vi "KenbakEngine.vi"(11 "Inputs":T11) -> (0 "Adder":T2, 1 "Clocks And Memory":T3, 2 "Control\nSignals":T7, 3 "States":T10, 4 "Instruction Specific":T1, 5 "K_reg":T6, 6 "W_reg":T4, 7 "I_reg":T5, 8 "L_reg":T8, 9 "T_reg":T9, 10 "Memory":cluster{"MemLo":u8, "MemHi":u8, "Carry?":bool} {"MemHi" format="%x"; "MemLo" format="%x"})   [LabVIEW 2012]
panel:
  out "JS4":bool
  out "JS3":bool
  out "JS2":bool
  out "JS1":bool
  out "JS0":bool
  out "JDL1":bool
  out "JDL0":bool
  out "KP":bool
  out "PF":bool
  out "PT":bool
  out "PO":bool
  out "ED":bool
  out "WD":bool
  out "BM":bool
  out "WT":bool
  out "WL":bool
  out "WJ":bool
  out "WK":bool
  out "CY":bool
  out "OV":bool
  out "OF":bool
  out "CR":bool
  out "SUM":bool
  out "ADD":bool
  out "C":bool
  out "JC":bool
  out "TS":bool
  out "BD":bool
  out "B":bool
  out "A":bool
  out "LONGLOGIC":bool
  out "LS":bool
  out "RR":bool
  out "BT":bool
  out "TX":bool
  out "HF":bool
  out "JW3":bool
  out "JW7":bool
  out "W7":bool
  out "W6":bool
  out "W5":bool
  out "W4":bool
  out "W3":bool
  out "W2":bool
  out "W1":bool
  out "W0":bool
  out "K7":bool
  out "K6":bool
  out "K5":bool
  out "K4":bool
  out "K3":bool
  out "K2":bool
  out "K1":bool
  out "K0":bool
  out "KS":bool
  out "Run":bool
  out "Input":bool
  out "Mem":bool
  out "Add":bool
  out "X4":bool
  out "X3":bool
  out "X2":bool
  out "X1":bool
  out "BU":bool
  out "MR":bool
  out "FT":bool
  out "I4":bool
  out "I5":bool
  out "I6":bool
  out "I7":bool
  out "I3":bool
  out "I2":bool
  out "I1":bool
  out "I0":bool
  out "CL":bool
  out "DA":bool
  out "HT":bool
  out "EA":bool
  out "DD":bool
  out "EN":bool
  out "GO":bool
  out "UT":bool
  out "IN":bool
  out "R":bool
  out "A7":bool
  out "SQ":bool
  out "SP":bool
  out "SW":bool
  out "SC":bool
  out "SD":bool
  out "SZ":bool
  out "SG":bool
  out "SM":bool
  out "SH":bool
  out "SK":bool
  out "SF":bool
  out "SN":bool
  out "SJ":bool
  out "SL":bool
  out "SA":bool
  out "QB":bool
  out "SX":bool
  out "SY":bool
  out "SB":bool
  out "ST":bool
  out "SV":bool
  out "SE":bool
  out "SU":bool
  out "SS":bool
  out "SR":bool
  out "QE":bool
  out "QF":bool
  out "QD":bool
  out "QC":bool
  out "Carry?":bool
  out "/ T7 \\":bool
  out "LC":bool
  out "CM":bool
  out "L7":bool
  out "L6":bool
  out "L5":bool
  out "L4":bool
  out "L3":bool
  out "L2":bool
  out "L1":bool
  out "L0":bool
  out "T7":bool
  out "T6":bool
  out "T5":bool
  out "T4":bool
  out "T3":bool
  out "T2":bool
  out "T1":bool
  out "T0":bool
  out "F1":bool
  out "F2":bool
  out "C7":bool
  out "CP":bool
  out "CT":bool
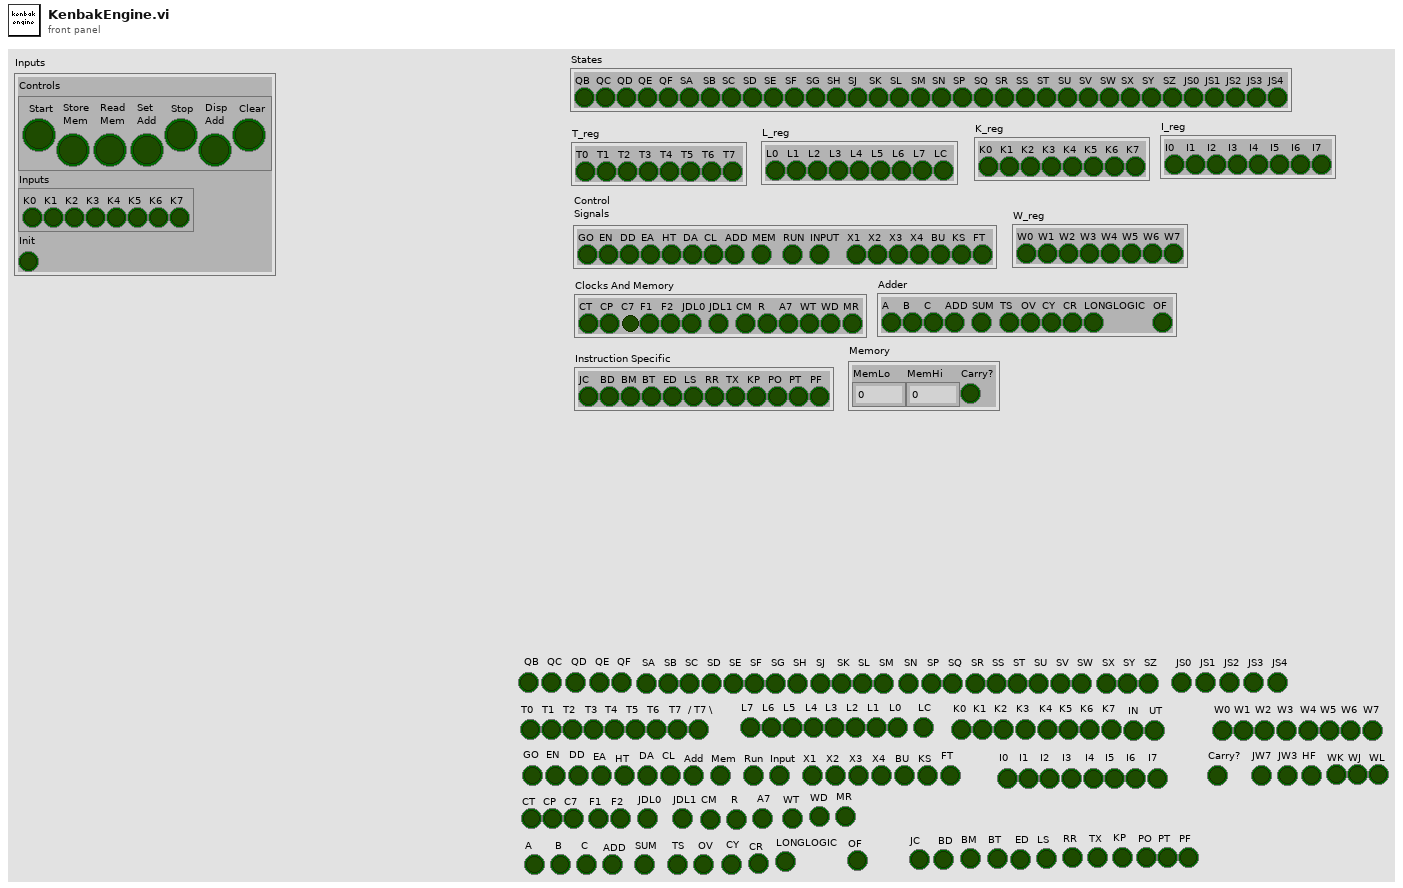
[diagram p1: front panel]
types:
  T1 = cluster{"JC":bool, "BD":bool, "BM":bool, "BT":bool, "ED":bool, "LS":bool, "RR":bool, "TX":bool, "KP":bool, "PO":bool, "PT":bool, "PF":bool}
  T2 = cluster{"A":bool, "B":bool, "C":bool, "ADD":bool, "SUM":bool, "TS":bool, "OV":bool, "CY":bool, "CR":bool, "LONGLOGIC":bool, "OF":bool}
  T3 = cluster{"CT":bool, "CP":bool, "C7":bool, "F1":bool, "F2":bool, "JDL0":bool, "JDL1":bool, "CM":bool, "R":bool, "A7":bool, "WT":bool, "WD":bool, "MR":bool}
  T4 = cluster{"W0":bool, "W1":bool, "W2":bool, "W3":bool, "W4":bool, "W5":bool, "W6":bool, "W7":bool}
  T5 = cluster{"I0":bool, "I1":bool, "I2":bool, "I3":bool, "I4":bool, "I5":bool, "I6":bool, "I7":bool}
  T6 = cluster{"K0":bool, "K1":bool, "K2":bool, "K3":bool, "K4":bool, "K5":bool, "K6":bool, "K7":bool}
  T7 = cluster{"GO":bool, "EN":bool, "DD":bool, "EA":bool, "HT":bool, "DA":bool, "CL":bool, "ADD":bool, "MEM":bool, "RUN":bool, "INPUT":bool, "X1":bool, "X2":bool, "X3":bool, "X4":bool, "BU":bool, "KS":bool, "FT":bool}
  T8 = cluster{"L0":bool, "L1":bool, "L2":bool, "L3":bool, "L4":bool, "L5":bool, "L6":bool, "L7":bool, "LC":bool}
  T9 = cluster{"T0":bool, "T1":bool, "T2":bool, "T3":bool, "T4":bool, "T5":bool, "T6":bool, "T7":bool}
  T10 = cluster{"QB":bool, "QC":bool, "QD":bool, "QE":bool, "QF":bool, "SA":bool, "SB":bool, "SC":bool, "SD":bool, "SE":bool, "SF":bool, "SG":bool, "SH":bool, "SJ":bool, "SK":bool, "SL":bool, "SM":bool, "SN":bool, "SP":bool, "SQ":bool, "SR":bool, "SS":bool, "ST":bool, "SU":bool, "SV":bool, "SW":bool, "SX":bool, "SY":bool, "SZ":bool, "JS0":bool, "JS1":bool, "JS2":bool, "JS3":bool, "JS4":bool}
  T11 = cluster{"Controls":cluster{"Start":bool, "Store\nMem":bool, "Read\nMem":bool, "Set\nAdd":bool, "Stop":bool, "Disp\nAdd":bool, "Clear":bool}, "Inputs":cluster{"K0":bool, "K1":bool, "K2":bool, "K3":bool, "K4":bool, "K5":bool, "K6":bool, "K7":bool}, "Init":bool}
  T12 = cluster{"Start":bool, "Store\nMem":bool, "Read\nMem":bool, "Set\nAdd":bool, "Stop":bool, "Disp\nAdd":bool, "Clear":bool}
  T13 = cluster{"OA":bool, "OB":bool, "OC":bool, "OD":bool, "OA":bool, "OB":bool, "OC":bool, "OD":bool}
  T14 = cluster{"OD":bool, "OC":bool, "OB":bool, "OA":bool, "OD":bool, "OC":bool, "OB":bool, "OA":bool, "Q":bool}
  T15 = cluster{"OA":bool, "OB":bool, "OC":bool, "OD":bool, bool, bool, bool, bool, bool, "0":bool, bool, bool, bool, bool, bool, bool, bool, bool}
  T16 = cluster{"1":bool, "0":bool, "1":bool, "3":bool, "2":bool, "0":bool, "4":bool, "2":bool, "3":bool, "7":bool, "3":bool, "7":bool, "1":bool, "5":bool, "2":bool, "6":bool, "0":bool, "4":bool, "0":bool, "6":bool, "4":bool, "5":bool, "5":bool, "6":bool, "6":bool, "1":bool, "2":bool, "3":bool, "4":bool, "Q":bool, "Q":bool, "Q":bool, "Q":bool, "Q":bool}
  T17 = cluster{"OD":bool, "OC":bool, "OB":bool, "OA":bool, "OD":bool, "OC":bool, "OB":bool, "OA":bool}
  T18 = cluster{bool, bool, "/Q\\":bool, bool, bool, "/Q\\":bool, "Q":bool, "Q":bool, bool, bool, bool}
  T19 = cluster{"Clk":bool, bool, bool, bool, bool, bool, bool, bool, bool, "/Q\\":bool, bool, bool, bool}
  T20 = cluster{bool, "Q":bool, bool, bool, "/Q\\":bool, bool, bool, "OD":bool, bool, "OD":bool, "OC":bool, "OB":bool}
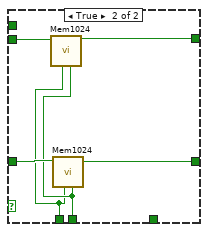
[diagram p2: hidden frame]
diagram:
  w204 = TRUE ("x")
  w226 = FALSE ("Serial\nInput")
  w257 = TRUE ("Set")
  w294 = TRUE ("Set")
  w295 = TRUE ("Set")
  w305 = FALSE ("y")
  w317 = TRUE ("Reset")
  w327 = TRUE ("Set")
  w338 = TRUE ("Set")
  w513 = TRUE ("Set")
  w514 = TRUE ("Set")
  w521 = TRUE ("Set")
  w638 = TRUE ("Set")
  w643 = TRUE ("Set")
  w650 = FALSE ("B")
  w651 = FALSE ("Mode\nControl")
  w654 = TRUE ("Set")
  w657 = FALSE ("B")
  w658 = FALSE ("Mode\nControl")
  w664 = TRUE
  w670 = TRUE ("Set")
  w672 = TRUE ("Set")
  # "JSX  0  1  2  3  4\nQB = 1, 0, 0, 1, 0\nQC = 0, 0, 0, 0, 0\nQD = 1, 0, 0, 0, 0\nQE = 1, 1, 0, 0, 0\nQF = 0, 1, 0, 0, 0\nSA = 0, 0, 0, 1, 0\nSB = 0, 0, 1, 1, 0\nSC = 0, 1, 0, 1, 1\nSD = 1, 1, 0, 1, 1\nSE = 1, 1, 1, 0, 0\nSF = 1, 1, 0, 0, 1\nSG = 1, 1, 1, 0, 1\nSH = 1, 0, 0, 0, 1\nSJ = 1, 0, 1, 0, 1\nSK = 0, 1, 0, 0, 1\nSL = 0, 1, 1, 0, 1\nSM = 0, 0, 0, 0, 1\nSN = 0, 0, 1, 0, 1\nSP = 0, 0, 0, 1, 1\nSQ = 0, 1, 1, 1, 1\nSR = 0, 0, 1, 0, 0\nSS = 1, 0, 1, 0, 0\nST = 1, 0, 1, 1, 0\nSU = 0, 1, 1, 0, 0\nSV = 0, 1, 1, 1, 0\nSW = 1, 0, 0, 1, 1\nSX = 0, 1, 0, 1, 0\nSY = 1, 1, 0, 1, 0\nSZ = 0, 0, 1, 1, 1"
  # "-IN+-BU"
  # "-IN+-CL"
  # "I11"
  # "I10"
  # "I2+-I1+I0"
  # "EN+DD"
  # "JS0"
  # "JS1"
  # "JS2"
  # "JS3"
  # "JS4"
  # "JS0B"
  # "JS0A"
  # "JS1B"
  # "JS2A"
  # "CM"
  # "JS1A"
  # "JS3A"
  # "JS3-4B"
  # "G5"
  # "G4"
  # "G3"
  # "G2"
  # "G1"
  n1 = Unbundle By Name("Inputs") -> ("Controls"=w165:T12)
  n2 = Unbundle By Name("Inputs") -> ("Inputs"=w2:T6)
  n3 = Unbundle By Name(w165) -> ("Start"=w164:bool, "Store\nMem"=w163:bool, "Read\nMem"=w162:bool, "Set\nAdd"=w161:bool, "Stop"=w106:bool, "Disp\nAdd"=w104:bool, "Clear"=w102:bool)
  n4 = Cluster To Array(cluster=w2) -> (array=w1:bool[])
  n5 = call "Clock.vi"("Slices"=u32 2) -> ("Clk"=w67:bool)  [unwired: 10 in]
  "CT" <- w67
  n6 = Index Array(array=w1) -> (element #1=w191:bool, element #2=w190:bool, element #3=w188:bool, element #4=w186:bool, element #5=w184:bool, element #6=w182:bool, element #7=w180:bool, element #8=w177:bool)  [unwired: 8 in]
  n7 = Not And(1:w67, 2:w67) -> (0:w673:bool)
  n8 = feedback #1() -> (w671:bool)  [unwired: 1 in]
  n9 = call "DflipFlop_Fast.vi"("D"=w671, "Clock"=w673, "Reset"=w672, "Set"=w672) -> ("/Q\\"=w175:bool, "Q"=w659:bool)  [unwired: 6 in]
  n10 = feedback-in #1(w175) -> ()
  n11 = Not(x=w182) -> (.not. x?=w181:bool)
  n12 = Not(x=w180) -> (.not. x?=w179:bool)
  n13 = Not(x=w177) -> (.not. x?=w178:bool)
  n14 = Not(x=w191) -> (.not. x?=w192:bool)
  n15 = Not(x=w190) -> (.not. x?=w189:bool)
  n16 = Not(x=w188) -> (.not. x?=w187:bool)
  n17 = Not(x=w186) -> (.not. x?=w185:bool)
  n18 = Not(x=w184) -> (.not. x?=w183:bool)
  n19 = feedback #2() -> (w640:bool)  [unwired: 1 in]
  n20 = Not(x=w106) -> (.not. x?=w105:bool)
  "HT" <- w105
  n21 = Not(x=w164) -> (.not. x?=w520:bool)
  n22 = Not(x=w162) -> (.not. x?=w518:bool)
  n23 = Not(x=w161) -> (.not. x?=w517:bool)
  n24 = Not(x=w104) -> (.not. x?=w103:bool)
  "DA" <- w103
  n25 = Not(x=w102) -> (.not. x?=w101:bool)
  "CL" <- w101
  n26 = Not(x=w163) -> (.not. x?=w519:bool)
  n27 = feedback #3() -> (w667:bool)  [unwired: 1 in]
  n28 = Compound Arithmetic op=AND(w667, w667, w640) -> (w669:bool)
  n29 = Not(x=w669) -> (.not. x?=w668:bool)
  n30 = call "DflipFlop_Fast.vi"("D"=w668, "Clock"=w659, "Reset"=w670, "Set"=w670) -> ("/Q\\"=w663:bool, "Q"=w662:bool)  [unwired: 6 in]
  n31 = feedback-in #3(w662) -> ()
  n32 = Not And(1:w659, 2:w659) -> (0:w661:bool)
  n33 = feedback #4() -> (w9:bool)  [unwired: 1 in]
  n34 = call "ReverseNot.vi"("In"=w9) -> ("~In"=w8:bool)  [unwired: 14 in]
  n35 = Not And(1:w8, 2:w659) -> (0:w660:bool)
  n36 = Not And(1:w8, 2:w8) -> (0:w639:bool)
  "/ T7 \\" <- w639
  n37 = feedback-in #2(w639) -> ()
  n38 = Not(x=w661) -> (.not. x?=w66:bool)
  "CP" <- w66
  n39 = call "7495_Fast2.vi"("Clk 1\nR-Shift"=w66, "Serial\nInput"=w8, "Clk 2\nL-Shift"=w66, "Mode\nControl"=w658, "D"=w658, "C"=w658, "B"=w658, "A"=w658) -> ("OD"=w12:bool, "OC"=w123:bool, "OB"=w124:bool, "OA"=w125:bool)
  "T0" <- w125
  "T1" <- w124
  "T2" <- w123
  "T3" <- w12
  n40 = Not And(1:w192, 2:w125) -> (0:w469:bool)
  n41 = Not And(1:w189, 2:w124) -> (0:w468:bool)
  n42 = Not And(1:w187, 2:w123) -> (0:w467:bool)
  n43 = Not And(1:w185, 2:w12) -> (0:w466:bool)
  n44 = Not(x=w660) -> (.not. x?=w65:bool)
  "C7" <- w65
  n45 = Not And(1:w65, 2:w65) -> (0:w555:bool)
  n46 = call "7495_Fast2.vi"("Clk 1\nR-Shift"=w66, "Serial\nInput"=FALSE ("Serial\nInput"), "Clk 2\nL-Shift"=w66, "Mode\nControl"=w12, "D"=w657, "C"=w657, "B"=w657, "A"=w12) -> ("OD"=w11:bool, "OC"=w120:bool, "OB"=w121:bool, "OA"=w122:bool)
  "T4" <- w122
  "T5" <- w121
  "T6" <- w120
  "T7" <- w11
  n47 = Not And(1:w183, 2:w122) -> (0:w465:bool)
  n48 = call "ReverseNot.vi"("In"=w11) -> ("~In"=w10:bool)  [unwired: 14 in]
  n49 = feedback-in #4(w10) -> ()
  n50 = Not And(1:w65, 2:w65) -> (0:w512:bool)
  n51 = feedback #5() -> (w457:bool)  [unwired: 1 in]
  n52 = feedback #6() -> (w456:bool)  [unwired: 1 in]
  n53 = Not And(1:w181, 2:w121) -> (0:w464:bool)
  n54 = Compound Arithmetic op=AND(w663, w664, w175) -> (w665:bool)
  n55 = Compound Arithmetic op=AND(w664, w175, w662) -> (w666:bool)
  n56 = Not(x=w665) -> (.not. x?=w64:bool)
  "F1" <- w64
  n57 = Not(x=w666) -> (.not. x?=w63:bool)
  "F2" <- w63
  n58 = feedback #7() -> (w511:bool)  [unwired: 1 in]
  n59 = call "DflipFlop_Fast.vi"("D"=w511, "Clock"=w512, "Reset"=w514, "Set"=w514) -> ("Q"=w445:bool)  [unwired: 6 in, 1 out]
  "UT" <- w445
  n60 = Not And(1:w179, 2:w120) -> (0:w463:bool)
  n61 = Exclusive Or(1:w66, 2:TRUE ("x")) -> (0:w642:bool)
  n62 = Not And(1:w178, 2:w11) -> (0:w462:bool)
  n63 = Compound Arithmetic op=AND(w101, w101, w101) -> (w210:bool)
  n64 = Not(x=w210) -> (.not. x?=w209:bool)
  n65 = Compound Arithmetic op=AND(w469, w468, w467, w466, w465, w464, w463, w462) -> (w96:bool)
  "BU" <- w96
  n66 = Not And(1:w96, 2:w96) -> (0:w174:bool)
  n67 = feedback #8() -> (w648:bool)  [unwired: 1 in]
  n68 = Bundle("OA"=w125, "OB"=w124, "OC"=w123, "OD"=w12, "OA"=w122, "OB"=w121, "OC"=w120, "OD"=w11) -> (→"T_reg":T13)  [unwired: 1 in]
  n69 = feedback #9() -> (w4:bool)  [unwired: 1 in]
  n70 = call "ReverseNot.vi"("In"=w4) -> ("~In"=w3:bool)  [unwired: 14 in]
  n71 = Not And(1:w3, 2:w648) -> (0:w653:bool)
  n72 = Not And(1:w639, 2:w653) -> (0:w652:bool)
  n73 = Exclusive Or(1:w3, 2:w648) -> (0:w649:bool)
  n74 = call "7495_Fast2.vi"("Clk 1\nR-Shift"=w66, "Serial\nInput"=w649, "Clk 2\nL-Shift"=w66, "Mode\nControl"=w651, "D"=w651, "C"=w651, "A"=w3) -> ("OD"=w7:bool, "OC"=w115:bool, "OB"=w114:bool, "OA"=w113:bool)  [unwired: 1 in]
  "L7" <- w113
  "L6" <- w114
  "L5" <- w115
  "L4" <- w7
  n75 = call "DflipFlop_Fast.vi"("D"=w652, "Clock"=w642, "Reset"=w654, "Set"=w654) -> ("Q"=w92:bool)  [unwired: 6 in, 1 out]
  "LC" <- w92
  n76 = call "DflipFlop.vi"("D"=w92, "Clock"=w512, "Reset"=w513, "Set"=w513) -> ("Q"=w207:bool)  [unwired: 6 in, 1 out]
  "IN" <- w207
  n77 = call "7495_Fast2.vi"("Clk 1\nR-Shift"=w207, "Serial\nInput"=FALSE ("Serial\nInput"), "Clk 2\nL-Shift"=w207, "Mode\nControl"=TRUE ("Mode\nControl"), "D"=w517, "C"=w518, "B"=w519, "A"=w520) -> ("OD"=w108:bool, "OC"=w109:bool, "OB"=w110:bool, "OA"=w111:bool)
  "GO" <- w111
  "EN" <- w110
  "DD" <- w109
  "EA" <- w108
  n78 = Not And(1:w111, 2:w111) -> (0:w193:bool)
  n79 = Compound Arithmetic op=AND(w103, w109, w457) -> (w460:bool)
  n80 = Compound Arithmetic op=AND(w110, w109, w103, w103) -> (w510:bool)
  n81 = Compound Arithmetic op=AND(w110, w109, w109, w110) -> (w509:bool)
  n82 = Not(x=w460) -> (.not. x?=w455:bool)
  n83 = Not(x=w510) -> (.not. x?=w508:bool)
  n84 = Not(x=w509) -> (.not. x?=w350:bool)
  n85 = feedback-in #7(w207) -> ()
  n86 = Not And(1:w209, 2:w207) -> (0:w208:bool)
  n87 = Not And(1:w96, 2:w207) -> (0:w206:bool)
  n88 = feedback-in #8(w92) -> ()
  n89 = And(x=w11, y=w92) -> (x .and. y?=w16:bool)
  "Carry?" <- w16
  n90 = Not And(1:w108, 2:w108) -> (0:w422:bool)
  n91 = call "7495_Fast2.vi"("Clk 1\nR-Shift"=w66, "Serial\nInput"=w7, "Clk 2\nL-Shift"=w66, "Mode\nControl"=w650, "D"=w66, "C"=w3, "B"=w650, "A"=w650) -> ("OD"=w5:bool, "OC"=w118:bool, "OB"=w117:bool, "OA"=w116:bool)
  "L3" <- w116
  "L2" <- w117
  "L1" <- w118
  "L0" <- w5
  n92 = call "ReverseNot.vi"("In"=w5) -> ("~In"=w6:bool)  [unwired: 14 in]
  n93 = feedback-in #9(w6) -> ()
  n94 = feedback #10() -> (w437:bool)  [unwired: 1 in]
  n95 = feedback #11() -> (w438:bool)  [unwired: 1 in]
  n96 = feedback #12() -> (w439:bool)  [unwired: 1 in]
  n97 = feedback #13() -> (w440:bool)  [unwired: 1 in]
  n98 = feedback #14() -> (w647:bool)  [unwired: 1 in]
  n99 = feedback #15() -> (w500:bool)  [unwired: 1 in]
  n100 = feedback #16() -> (w501:bool)  [unwired: 1 in]
  n101 = feedback #17() -> (w502:bool)  [unwired: 1 in]
  n102 = feedback #18() -> (w503:bool)  [unwired: 1 in]
  n103 = Bundle("OD"=w5, "OC"=w118, "OB"=w117, "OA"=w116, "OD"=w7, "OC"=w115, "OB"=w114, "OA"=w113, "Q"=w92) -> (→"L_reg":T14)  [unwired: 1 in]
  n104 = feedback #19() -> (w444:bool)  [unwired: 1 in]
  n105 = feedback #20() -> (w443:bool)  [unwired: 1 in]
  n106 = feedback #21() -> (w442:bool)  [unwired: 1 in]
  n107 = feedback #22() -> (w441:bool)  [unwired: 1 in]
  n108 = feedback #23() -> (w507:bool)  [unwired: 1 in]
  n109 = feedback #24() -> (w506:bool)  [unwired: 1 in]
  n110 = feedback #25() -> (w505:bool)  [unwired: 1 in]
  n111 = feedback #26() -> (w504:bool)  [unwired: 1 in]
  n112 = Not And(1:w125, 2:w125) -> (0:w379:bool)
  n113 = Not And(1:w122, 2:w122) -> (0:w369:bool)
  n114 = feedback #27() -> (w381:bool)  [unwired: 1 in]
  n115 = feedback #28() -> (w554:bool)  [unwired: 1 in]
  n116 = call "DflipFlop_Fast.vi"("D"=w554, "Clock"=w555, "Reset"=w638, "Set"=w638) -> ("Q"=w131:bool)  [unwired: 6 in, 1 out]
  "JS0" <- w131
  n117 = feedback #29() -> (w553:bool)  [unwired: 1 in]
  n118 = call "DflipFlop_Fast.vi"("D"=w553, "Clock"=w555, "Reset"=w638, "Set"=w638) -> ("Q"=w130:bool)  [unwired: 6 in, 1 out]
  "JS1" <- w130
  n119 = feedback #30() -> (w552:bool)  [unwired: 1 in]
  n120 = call "DflipFlop_Fast.vi"("D"=w552, "Clock"=w555, "Reset"=w638, "Set"=w638) -> ("Q"=w129:bool)  [unwired: 6 in, 1 out]
  "JS2" <- w129
  n121 = feedback #31() -> (w551:bool)  [unwired: 1 in]
  n122 = call "DflipFlop_Fast.vi"("D"=w551, "Clock"=w555, "Reset"=w638, "Set"=w638) -> ("/Q\\"=w636:bool, "Q"=w128:bool)  [unwired: 6 in]
  "JS3" <- w128
  n123 = feedback #32() -> (w550:bool)  [unwired: 1 in]
  n124 = call "DflipFlop_Fast.vi"("D"=w550, "Clock"=w555, "Reset"=w638, "Set"=w638) -> ("/Q\\"=w637:bool, "Q"=w127:bool)  [unwired: 6 in]
  "JS4" <- w127
  n125 = Not And(1:w637, 2:w636) -> (0:w632:bool)
  n126 = Not And(1:w637, 2:w128) -> (0:w633:bool)
  n127 = Not And(1:w127, 2:w636) -> (0:w634:bool)
  n128 = Not And(1:w127, 2:w128) -> (0:w635:bool)
  n129 = call "7442.vi"("D"=w635, "C"=w129, "B"=w130, "A"=w131) -> ("0"=w142:bool, "1"=w135:bool, "2"=w153:bool, "3"=w152:bool, "4"=w132:bool, "6"=w141:bool)  [unwired: 2 in, 4 out]
  "SP" <- w142
  "SW" <- w135
  "SC" <- w153
  "SD" <- w152
  "SZ" <- w132
  "SQ" <- w141
  n130 = call "7442.vi"("D"=w632, "C"=w129, "B"=w130, "A"=w131) -> ("0"=w107:bool, "1"=w158:bool, "2"=w156:bool, "3"=w157:bool, "4"=w139:bool, "5"=w140:bool, "6"=w137:bool, "7"=w151:bool)  [unwired: 2 in, 2 out]
  "QC" <- w107
  "QD" <- w158
  "QF" <- w156
  "QE" <- w157
  "SR" <- w139
  "SS" <- w140
  "SU" <- w137
  "SE" <- w151
  "Run" <- w107
  n131 = call "7442.vi"("D"=w633, "C"=w129, "B"=w130, "A"=w131) -> ("0"=w155:bool, "1"=w159:bool, "2"=w134:bool, "3"=w133:bool, "4"=w154:bool, "5"=w138:bool, "6"=w136:bool)  [unwired: 2 in, 3 out]
  "SA" <- w155
  "QB" <- w159
  "SX" <- w134
  "SY" <- w133
  "SB" <- w154
  "ST" <- w138
  "SV" <- w136
  n132 = Compound Arithmetic op=AND(w455, w155, w101, w174) -> (w461:bool)
  n133 = Compound Arithmetic op=AND(w103, w155, w456) -> (w459:bool)
  n134 = Not(x=w461) -> (.not. x?=w453:bool)
  n135 = feedback-in #5(w453) -> ()
  n136 = Not(x=w459) -> (.not. x?=w454:bool)
  n137 = Compound Arithmetic op=AND(w454, w109, w101, w174) -> (w458:bool)
  n138 = Not(x=w458) -> (.not. x?=w452:bool)
  n139 = feedback-in #6(w452) -> ()
  n140 = And(x=w454, y=w455) -> (x .and. y?=w100:bool)
  "X1" <- w100
  "Add" <- w100
  n141 = And(x=w455, y=w452) -> (x .and. y?=w99:bool)
  "X2" <- w99
  "Mem" <- w99
  n142 = And(x=w454, y=w453) -> (x .and. y?=w98:bool)
  "X3" <- w98
  n143 = And(x=w453, y=w452) -> (x .and. y?=w97:bool)
  "X4" <- w97
  "Input" <- w97
  n144 = call "7442.vi"("D"=w634, "C"=w129, "B"=w130, "A"=w131) -> ("0"=w144:bool, "1"=w148:bool, "2"=w146:bool, "3"=w150:bool, "4"=w143:bool, "5"=w147:bool, "6"=w145:bool, "7"=w149:bool)  [unwired: 2 in, 2 out]
  "SM" <- w144
  "SH" <- w148
  "SK" <- w146
  "SF" <- w150
  "SN" <- w143
  "SJ" <- w147
  "SL" <- w145
  "SG" <- w149
  n145 = Not And(1:w157, 2:w157) -> (0:w446:bool)
  n146 = And(x=w446, y=w99) -> (x .and. y?=w447:bool)
  n147 = And(x=w446, y=w100) -> (x .and. y?=w448:bool)
  n148 = And(x=w207, y=w97) -> (x .and. y?=w449:bool)
  n149 = And(x=w98, y=w445) -> (x .and. y?=w450:bool)
  n150 = Compound Arithmetic op=OR(w447, w448, w449, w450) -> (w451:bool)
  n151 = Not(x=w451) -> (.not. x?=w95:bool)
  "KS" <- w95
  n152 = Not And(1:w107, 2:w107) -> (0:w498:bool)
  n153 = Not And(1:w207, 2:w498) -> (0:w424:bool)
  n154 = Not And(1:w424, 2:w424) -> (0:w423:bool)
  n155 = Compound Arithmetic op=AND(w152, w141, w157, w140, w424, w424, w142, w157) -> (w499:bool)
  n156 = Not(x=w499) -> (.not. x?=w94:bool)
  "FT" <- w94
  n157 = Bundle("OA"=w111, "OB"=w110, "OC"=w109, "OD"=w108, w105, w103, w101, w100, w99, "0"=w107, w97, w100, w99, w98, w97, w96, w95, w94) -> (→"Control\nSignals":T15)  [unwired: 1 in]
  n158 = Not And(1:w422, 2:w423) -> (0:w421:bool)
  n159 = Not And(1:w94, 2:w94) -> (0:w172:bool)
  n160 = Bundle("1"=w159, "0"=w107, "1"=w158, "3"=w157, "2"=w156, "0"=w155, "4"=w154, "2"=w153, "3"=w152, "7"=w151, "3"=w150, "7"=w149, "1"=w148, "5"=w147, "2"=w146, "6"=w145, "0"=w144, "4"=w143, "0"=w142, "6"=w141, "4"=w139, "5"=w140, "5"=w138, "6"=w137, "6"=w136, "1"=w135, "2"=w134, "3"=w133, "4"=w132, "Q"=w131, "Q"=w130, "Q"=w129, "Q"=w128, "Q"=w127) -> (→"States":T16)  [unwired: 1 in]
  n161 = Not(x=w144) -> (.not. x?=w195:bool)
  n162 = Not(x=w158) -> (.not. x?=w611:bool)
  n163 = Not(x=w154) -> (.not. x?=w630:bool)
  n164 = Not(x=w138) -> (.not. x?=w196:bool)
  n165 = Not(x=w145) -> (.not. x?=w263:bool)
  n166 = Not And(1:w151, 2:w151) -> (0:w352:bool)
  n167 = Not And(1:w156, 2:w156) -> (0:w610:bool)
  n168 = Not And(1:w149, 2:w149) -> (0:w194:bool)
  n169 = Not And(1:w107, 2:w107) -> (0:w544:bool)
  n170 = Not And(1:w132, 2:w132) -> (0:w623:bool)
  n171 = Not And(1:w136, 2:w136) -> (0:w253:bool)
  n172 = Compound Arithmetic op=AND(w152, w152, w137, w137) -> (w628:bool)
  n173 = Not(x=w628) -> (.not. x?=w627:bool)
  n174 = Not And(1:w627, 2:w627) -> (0:w564:bool)
  n175 = Not And(1:w137, 2:w134) -> (0:w532:bool)
  n176 = And(x=w193, y=w544) -> (x .and. y?=w621:bool)
  n177 = Not And(1:w144, 2:w144) -> (0:w529:bool)
  n178 = feedback #33() -> (w378:bool)  [unwired: 1 in]
  n179 = Not And(1:w378, 2:w379) -> (0:w377:bool)
  n180 = Not And(1:w369, 2:w377) -> (0:w376:bool)
  n181 = feedback-in #33(w376) -> ()
  n182 = feedback #34() -> (w387:bool)  [unwired: 1 in]
  n183 = And(x=w610, y=w508) -> (x .and. y?=w614:bool)
  n184 = Compound Arithmetic op=AND(w147, w144, w151, w149) -> (w583:bool)
  n185 = Compound Arithmetic op=AND(w152, w153, w150, w158, w139, w146, w146, w139) -> (w534:bool)
  n186 = Not(x=w583) -> (.not. x?=w582:bool)
  n187 = Not(x=w534) -> (.not. x?=w524:bool)
  n188 = Not And(1:w135, 2:w135) -> (0:w400:bool)
  n189 = Not And(1:w582, 2:w582) -> (0:w584:bool)
  n190 = Not And(1:w107, 2:w107) -> (0:w523:bool)
  n191 = And(x=w107, y=FALSE) -> (x .and. y?=w541:bool)
  n192 = Compound Arithmetic op=AND(w157, w151, w154, w149, w145, w136, w421, w147) -> (w425:bool)
  n193 = Not And(1:w152, 2:w152) -> (0:w248:bool)
  n194 = Not And(1:w159, 2:w159) -> (0:w593:bool)
  n195 = And(x=w523, y=w523) -> (x .and. y?=w526:bool)
  n196 = Not(x=w425) -> (.not. x?=w414:bool)
  n197 = feedback #35() -> (w371:bool)  [unwired: 1 in]
  n198 = And(x=w593, y=w193) -> (x .and. y?=w594:bool)
  n199 = And(x=w544, y=w508) -> (x .and. y?=w597:bool)
  n200 = Not And(1:w193, 2:w544) -> (0:w590:bool)
  n201 = Not And(1:w414, 2:w414) -> (0:w417:bool)
  n202 = Compound Arithmetic op=AND(w140, w133, w136, w143, w143, w132, w132, w132) -> (w578:bool)
  n203 = Not(x=w578) -> (.not. x?=w577:bool)
  n204 = Not And(1:w66, 2:w66) -> (0:w313:bool)
  n205 = Not And(1:w11, 2:w11) -> (0:w316:bool)
  n206 = Not And(1:w577, 2:w577) -> (0:w576:bool)
  n207 = Not And(1:w65, 2:w65) -> (0:w293:bool)
  n208 = Compound Arithmetic op=AND(w148, w146, w150, w155) -> (w572:bool)
  n209 = Not(x=w572) -> (.not. x?=w571:bool)
  n210 = feedback #36() -> (w335:bool)  [unwired: 1 in]
  n211 = Compound Arithmetic op=AND(w139, w134, w153, w153) -> (w543:bool)
  n212 = Not(x=w543) -> (.not. x?=w561:bool)
  n213 = feedback #37() -> (w394:bool)  [unwired: 1 in]
  n214 = feedback #38() -> (w426:bool)  [unwired: 1 in]
  n215 = feedback #39() -> (w427:bool)  [unwired: 1 in]
  n216 = feedback #40() -> (w395:bool)  [unwired: 1 in]
  n217 = Not And(1:w157, 2:w157) -> (0:w351:bool)
  n218 = feedback #41() -> (w430:bool)  [unwired: 1 in]
  n219 = feedback #42() -> (w429:bool)  [unwired: 1 in]
  n220 = feedback #43() -> (w428:bool)  [unwired: 1 in]
  n221 = feedback #44() -> (w393:bool)  [unwired: 1 in]
  n222 = And(x=w100, y=w393) -> (x .and. y?=w436:bool)
  n223 = And(x=w393, y=w524) -> (x .and. y?=w528:bool)
  n224 = And(x=w524, y=w393) -> (x .and. y?=w525:bool)
  n225 = Not Or(1:w526, 2:w525) -> (0:w522:bool)
  n226 = call "DflipFlop_Fast.vi"("D"=w522, "Clock"=w65, "Reset"=w521, "Set"=w521) -> ("/Q\\"=w58:bool, "Q"=w171:bool)  [unwired: 6 in]
  "A7" <- w58
  n227 = Not And(1:w151, 2:w151) -> (0:w353:bool)
  n228 = Not And(1:w143, 2:w143) -> (0:w283:bool)
  n229 = Not And(1:w350, 2:w351) -> (0:w347:bool)
  n230 = Not And(1:w154, 2:w154) -> (0:w341:bool)
  n231 = Not And(1:w141, 2:w141) -> (0:w339:bool)
  n232 = Not And(1:w11, 2:w11) -> (0:w315:bool)
  n233 = And(x=w124, y=w339) -> (x .and. y?=w357:bool)
  n234 = Not And(1:w105, 2:w105) -> (0:w167:bool)
  n235 = Not And(1:w141, 2:w133) -> (0:w287:bool)
  n236 = Not And(1:w110, 2:w110) -> (0:w280:bool)
  n237 = Not And(1:w157, 2:w157) -> (0:w279:bool)
  n238 = Not And(1:w287, 2:w287) -> (0:w284:bool)
  n239 = Not And(1:w280, 2:w279) -> (0:w278:bool)
  n240 = Not And(1:w278, 2:w140) -> (0:w259:bool)
  "WL" <- w259
  n241 = And(x=w259, y=w259) -> (x .and. y?=w275:bool)
  n242 = Not And(1:TRUE ("y"), 2:w66) -> (0:w245:bool)
  n243 = feedback #45() -> (w311:bool)  [unwired: 1 in]
  n244 = call "7495_Fast2.vi"("Clk 1\nR-Shift"=w66, "Serial\nInput"=w311, "Clk 2\nL-Shift"=w66, "Mode\nControl"=w172, "D"=w503, "C"=w502, "B"=w501, "A"=w500) -> ("OD"=w15:bool, "OC"=w80:bool, "OB"=w79:bool, "OA"=w78:bool)
  "I4" <- w15
  "I5" <- w80
  "I6" <- w79
  "I7" <- w78
  n245 = feedback-in #15(w78) -> ()
  n246 = feedback-in #16(w79) -> ()
  n247 = feedback-in #17(w80) -> ()
  n248 = feedback-in #18(w15) -> ()
  n249 = call "7495_Fast2.vi"("Clk 1\nR-Shift"=w66, "Serial\nInput"=w15, "Clk 2\nL-Shift"=w66, "Mode\nControl"=w172, "D"=w504, "C"=w505, "B"=w506, "A"=w507) -> ("OD"=w84:bool, "OC"=w83:bool, "OB"=w82:bool, "OA"=w81:bool)
  "I0" <- w84
  "I1" <- w83
  "I2" <- w82
  "I3" <- w81
  n250 = feedback-in #23(w81) -> ()
  n251 = feedback-in #24(w82) -> ()
  n252 = feedback-in #25(w83) -> ()
  n253 = feedback-in #26(w84) -> ()
  n254 = Not(x=w80) -> (.not. x?=w282:bool)
  n255 = Not And(1:w15, 2:w15) -> (0:w492:bool)
  n256 = Not(x=w84) -> (.not. x?=w485:bool)
  n257 = Not And(1:w82, 2:w82) -> (0:w484:bool)
  n258 = Compound Arithmetic op=AND(w484, w485, w83) -> (w491:bool)
  n259 = Not And(1:w84, 2:w253) -> (0:w557:bool)
  n260 = Not(x=w491) -> (.not. x?=w267:bool)
  n261 = Not And(1:w263, 2:w267) -> (0:w581:bool)
  n262 = Not And(1:w263, 2:w581) -> (0:w574:bool)
  n263 = Not And(1:w83, 2:w83) -> (0:w481:bool)
  n264 = Not And(1:w84, 2:w84) -> (0:w480:bool)
  n265 = Not(x=w79) -> (.not. x?=w239:bool)
  n266 = Not And(1:w79, 2:w78) -> (0:w366:bool)
  n267 = Not And(1:w81, 2:w15) -> (0:w389:bool)
  n268 = Not And(1:w78, 2:w78) -> (0:w266:bool)
  n269 = Not And(1:w282, 2:w282) -> (0:w486:bool)
  n270 = Not And(1:w480, 2:w481) -> (0:w482:bool)
  n271 = Not(x=w366) -> (.not. x?=w495:bool)
  n272 = Not(x=w366) -> (.not. x?=w290:bool)
  n273 = Not And(1:w82, 2:w82) -> (0:w365:bool)
  n274 = Not And(1:w81, 2:w81) -> (0:w388:bool)
  n275 = Not And(1:w495, 2:w389) -> (0:w349:bool)
  n276 = Not(x=w389) -> (.not. x?=w494:bool)
  n277 = Compound Arithmetic op=AND(w282, w84, w82) -> (w488:bool)
  n278 = Compound Arithmetic op=AND(w482, w282, w82) -> (w483:bool)
  n279 = Compound Arithmetic op=AND(w267, w486, w81) -> (w487:bool)
  n280 = Not And(1:w388, 2:w365) -> (0:w493:bool)
  n281 = Not And(1:w81, 2:w15) -> (0:w322:bool)
  n282 = Not And(1:w388, 2:w15) -> (0:w392:bool)
  n283 = Not And(1:w81, 2:w389) -> (0:w391:bool)
  n284 = Not And(1:w388, 2:w389) -> (0:w390:bool)
  n285 = Not And(1:w366, 2:w78) -> (0:w496:bool)
  n286 = Not And(1:w79, 2:w366) -> (0:w497:bool)
  n287 = Not(x=w488) -> (.not. x?=w476:bool)
  n288 = Not(x=w483) -> (.not. x?=w473:bool)
  n289 = Not(x=w487) -> (.not. x?=w475:bool)
  n290 = Not And(1:w494, 2:w366) -> (0:w489:bool)
  n291 = Not And(1:w489, 2:w282) -> (0:w603:bool)
  n292 = Compound Arithmetic op=AND(w489, w481, w282, w82) -> (w490:bool)
  n293 = Not(x=w490) -> (.not. x?=w477:bool)
  n294 = Not(x=w496) -> ()  [unwired: 1 out]
  n295 = Not(x=w497) -> (.not. x?=w472:bool)
  n296 = Not And(1:w489, 2:w489) -> (0:w169:bool)
  n297 = Not And(1:w169, 2:w282) -> (0:w545:bool)
  n298 = call "7495_Fast2.vi"("Clk 1\nR-Shift"=w66, "Serial\nInput"=w387, "Clk 2\nL-Shift"=w66, "Mode\nControl"=w11, "D"=w390, "C"=w391, "B"=w392, "A"=w322) -> ("OD"=w34:bool)  [unwired: 3 out]
  "TX" <- w34
  n299 = Compound Arithmetic op=AND(w477, w267, w476, w475) -> (w478:bool)
  n300 = Not(x=w282) -> (.not. x?=w479:bool)
  n301 = Not And(1:w473, 2:w475) -> (0:w168:bool)
  n302 = Not(x=w478) -> (.not. x?=w474:bool)
  n303 = feedback-in #34(w34) -> ()
  n304 = Compound Arithmetic op=AND(w194, w282, w481) -> (w600:bool)
  n305 = Not And(1:w34, 2:w34) -> (0:w372:bool)
  n306 = Compound Arithmetic op=AND(w372, w379, w372) -> (w386:bool)
  n307 = Not(x=w386) -> (.not. x?=w382:bool)
  n308 = Not And(1:w381, 2:w382) -> (0:w35:bool)
  "RR" <- w35
  n309 = Not And(1:w379, 2:w35) -> (0:w380:bool)
  n310 = feedback-in #27(w380) -> ()
  n311 = Not And(1:w80, 2:w80) -> (0:w323:bool)
  n312 = Not And(1:w529, 2:w472) -> (0:w531:bool)
  n313 = Not And(1:w479, 2:w532) -> (0:w533:bool)
  n314 = Not And(1:w472, 2:w529) -> (0:w530:bool)
  n315 = Not(x=w600) -> (.not. x?=w599:bool)
  n316 = And(x=w352, y=w474) -> (x .and. y?=w616:bool)
  n317 = Not And(1:w599, 2:w147) -> (0:w601:bool)
  n318 = Compound Arithmetic op=AND(w323, w372, w377) -> (w385:bool)
  n319 = Compound Arithmetic op=AND(w376, w372, w80) -> (w384:bool)
  n320 = Compound Arithmetic op=AND(w155, w148, w530, w138) -> (w536:bool)
  n321 = Compound Arithmetic op=AND(w155, w533, w531, w138) -> (w538:bool)
  n322 = Not(x=w385) -> (.not. x?=w374:bool)
  n323 = Not(x=w384) -> (.not. x?=w375:bool)
  n324 = Not(x=w536) -> (.not. x?=w535:bool)
  n325 = Not(x=w538) -> (.not. x?=w537:bool)
  n326 = Not And(1:w601, 2:w489) -> (0:w566:bool)
  n327 = Not(x=w78) -> (.not. x?=w403:bool)
  n328 = Compound Arithmetic op=AND(w372, w372, w369) -> (w373:bool)
  n329 = Compound Arithmetic op=AND(w374, w375, w375) -> (w383:bool)
  n330 = Not(x=w373) -> (.not. x?=w368:bool)
  n331 = And(x=w537, y=w125) -> (x .and. y?=w542:bool)
  n332 = And(x=w124, y=w535) -> (x .and. y?=w540:bool)
  n333 = Not(x=w383) -> (.not. x?=w38:bool)
  "BT" <- w38
  n334 = Compound Arithmetic op=AND(w400, w239, w403) -> (w420:bool)
  n335 = Not(x=w420) -> (.not. x?=w416:bool)
  n336 = Compound Arithmetic op=AND(w194, w481, w282) -> (w587:bool)
  n337 = Compound Arithmetic op=OR(w542, w541, w540, w528) -> (w539:bool)
  n338 = Not And(1:w35, 2:w35) -> (0:w404:bool)
  n339 = Not And(1:w371, 2:w368) -> (0:w370:bool)
  n340 = Not And(1:w369, 2:w370) -> (0:w36:bool)
  "LS" <- w36
  n341 = Compound Arithmetic op=AND(w78, w239, w36) -> (w419:bool)
  n342 = Not(x=w419) -> (.not. x?=w408:bool)
  n343 = feedback-in #35(w36) -> ()
  n344 = Not(x=w587) -> (.not. x?=w586:bool)
  n345 = And(x=w168, y=w352) -> (x .and. y?=w595:bool)
  n346 = And(x=w248, y=w493) -> (x .and. y?=w596:bool)
  n347 = Not(x=w539) -> (.not. x?=w59:bool)
  "R" <- w59
  n348 = Exclusive Or(1:w3, 2:w59) -> (0:w641:bool)
  n349 = Not And(1:w641, 2:w647) -> (0:w644:bool)
  n350 = Not And(1:w639, 2:w644) -> (0:w645:bool)
  n351 = call "DflipFlop_Fast.vi"("D"=w645, "Clock"=w642, "Reset"=w643, "Set"=w643) -> ("/Q\\"=w197:bool, "Q"=w646:bool)  [unwired: 6 in]
  n352 = feedback-in #14(w646) -> ()
  n353 = Not And(1:w197, 2:w197) -> (0:w60:bool)
  "CM" <- w60
  n354 = Compound Arithmetic op=AND(w60, w60, w60) -> (w617:bool)
  n355 = Not(x=w617) -> (.not. x?=w588:bool)
  n356 = Not And(1:w60, 2:w603) -> (0:w604:bool)
  n357 = Compound Arithmetic op=AND(w492, w60, w492) -> (w606:bool)
  n358 = Not And(1:w604, 2:w604) -> (0:w602:bool)
  n359 = Not(x=w606) -> (.not. x?=w605:bool)
  n360 = And(x=w532, y=w60) -> (x .and. y?=w618:bool)
  n361 = And(x=w195, y=w602) -> (x .and. y?=w619:bool)
  n362 = And(x=w605, y=w196) -> (x .and. y?=w620:bool)
  n363 = Not And(1:w60, 2:w196) -> (0:w580:bool)
  n364 = Not And(1:w60, 2:w196) -> (0:w608:bool)
  n365 = Compound Arithmetic op=OR(w618, w619, w620, w621) -> (w622:bool)
  n366 = Not And(1:w608, 2:w608) -> (0:w609:bool)
  n367 = Not(x=w622) -> (.not. x?=w575:bool)
  n368 = Compound Arithmetic op=AND(w195, w60, w545) -> (w607:bool)
  n369 = And(x=w611, y=w60) -> (x .and. y?=w615:bool)
  n370 = And(x=w15, y=w609) -> (x .and. y?=w613:bool)
  n371 = Not(x=w607) -> (.not. x?=w569:bool)
  n372 = Compound Arithmetic op=OR(w616, w615, w614, w613) -> (w612:bool)
  n373 = Not(x=w612) -> (.not. x?=w567:bool)
  n374 = Not And(1:w588, 2:w196) -> (0:w589:bool)
  n375 = Compound Arithmetic op=AND(w408, w408, w408) -> (w409:bool)
  n376 = Not And(1:w403, 2:w404) -> (0:w401:bool)
  n377 = Not And(1:w78, 2:w35) -> (0:w252:bool)
  n378 = Not And(1:w416, 2:w416) -> (0:w415:bool)
  n379 = Compound Arithmetic op=OR(w594, w595, w596, w597) -> (w598:bool)
  n380 = Not(x=w409) -> (.not. x?=w407:bool)
  n381 = Compound Arithmetic op=AND(w590, w586, w589) -> (w592:bool)
  n382 = Not(x=w592) -> (.not. x?=w591:bool)
  n383 = Not(x=w598) -> (.not. x?=w560:bool)
  n384 = Compound Arithmetic op=AND(w417, w416, w393) -> (w418:bool)
  n385 = Not And(1:w415, 2:w394) -> (0:w410:bool)
  n386 = Compound Arithmetic op=AND(w252, w401, w400) -> (w402:bool)
  n387 = Bundle("OD"=w84, "OC"=w83, "OB"=w82, "OA"=w81, "OD"=w15, "OC"=w80, "OB"=w79, "OA"=w78) -> (→"I_reg":T17)  [unwired: 1 in]
  n388 = Not And(1:w400, 2:w407) -> (0:w406:bool)
  n389 = Not And(1:w414, 2:w311) -> (0:w411:bool)
  n390 = Not And(1:w79, 2:w78) -> (0:w324:bool)
  n391 = Not(x=w418) -> (.not. x?=w412:bool)
  n392 = Not(x=w402) -> (.not. x?=w399:bool)
  n393 = Not And(1:w591, 2:w591) -> (0:w559:bool)
  n394 = Not And(1:w406, 2:w395) -> (0:w405:bool)
  n395 = Compound Arithmetic op=AND(w323, w322, w324, w283) -> (w326:bool)
  n396 = Not And(1:w399, 2:w399) -> (0:w396:bool)
  "HF" <- w396
  n397 = Compound Arithmetic op=AND(w412, w411, w410) -> (w413:bool)
  n398 = Not(x=w326) -> (.not. x?=w325:bool)
  n399 = Not And(1:w405, 2:w405) -> (0:w397:bool)
  "JW3" <- w397
  n400 = Not(x=w413) -> (.not. x?=w398:bool)
  "JW7" <- w398
  n401 = call "DflipFlop_Fast.vi"("D"=w325, "Clock"=w293, "Reset"=w327, "Set"=w327) -> ("/Q\\"=w48:bool, "Q"=w176:bool)  [unwired: 6 in]
  "TS" <- w48
  n402 = Not And(1:w571, 2:w60) -> (0:w570:bool)
  n403 = Not And(1:w561, 2:w60) -> (0:w558:bool)
  n404 = Not And(1:w83, 2:w83) -> (0:w319:bool)
  n405 = call "7495_Fast2.vi"("Clk 1\nR-Shift"=w66, "Serial\nInput"=w398, "Clk 2\nL-Shift"=w66, "Mode\nControl"=w396, "D"=w395, "C"=w427, "B"=w426, "A"=w394) -> ("OD"=w72:bool, "OC"=w71:bool, "OB"=w70:bool, "OA"=w69:bool)
  "W4" <- w72
  "W5" <- w71
  "W6" <- w70
  "W7" <- w69
  n406 = feedback-in #37(w69) -> ()
  n407 = feedback-in #38(w70) -> ()
  n408 = feedback-in #39(w71) -> ()
  n409 = feedback-in #40(w72) -> ()
  n410 = Compound Arithmetic op=AND(w83, w366, w282, w365, w366, w84, w15, w81) -> (w367:bool)
  n411 = Not And(1:w84, 2:w84) -> (0:w249:bool)
  n412 = Not And(1:w319, 2:w84) -> (0:w318:bool)
  n413 = Not(x=w367) -> (.not. x?=w364:bool)
  n414 = Not(x=w364) -> (.not. x?=w44:bool)
  "LONGLOGIC" <- w44
  n415 = call "7495_Fast2.vi"("Clk 1\nR-Shift"=w66, "Serial\nInput"=w397, "Clk 2\nL-Shift"=w66, "Mode\nControl"=w396, "D"=w393, "C"=w428, "B"=w429, "A"=w430) -> ("OD"=w76:bool, "OC"=w75:bool, "OB"=w74:bool, "OA"=w73:bool)
  "W0" <- w76
  "W1" <- w75
  "W2" <- w74
  "W3" <- w73
  n416 = feedback-in #41(w73) -> ()
  n417 = feedback-in #42(w74) -> ()
  n418 = feedback-in #43(w75) -> ()
  n419 = feedback-in #44(w76) -> ()
  n420 = Not And(1:w349, 2:w283) -> (0:w348:bool)
  n421 = Not And(1:w353, 2:w44) -> (0:w346:bool)
  n422 = Not(x=w81) -> (.not. x?=w289:bool)
  n423 = Not And(1:w347, 2:w346) -> (0:w340:bool)
  n424 = Not And(1:w348, 2:w147) -> (0:w342:bool)
  n425 = Not And(1:w346, 2:w157) -> (0:w344:bool)
  n426 = Not And(1:w15, 2:w283) -> (0:w354:bool)
  n427 = Compound Arithmetic op=AND(w344, w344, w344) -> (w363:bool)
  n428 = Not And(1:w267, 2:w267) -> (0:w264:bool)
  n429 = Not(x=w363) -> (.not. x?=w345:bool)
  n430 = Compound Arithmetic op=AND(w264, w38, w263) -> (w265:bool)
  n431 = Not(x=w265) -> (.not. x?=w262:bool)
  n432 = And(x=w125, y=w340) -> (x .and. y?=w359:bool)
  n433 = And(x=w76, y=w342) -> (x .and. y?=w358:bool)
  n434 = Compound Arithmetic op=AND(w76, w344, w344) -> (w361:bool)
  n435 = Not And(1:w262, 2:w262) -> (0:w39:bool)
  "BM" <- w39
  n436 = Not(x=w361) -> (.not. x?=w343:bool)
  n437 = Compound Arithmetic op=AND(w253, w252, w249) -> (w255:bool)
  n438 = And(x=w39, y=w266) -> (x .and. y?=w276:bool)
  n439 = And(x=w259, y=w84) -> (x .and. y?=w269:bool)
  n440 = And(x=w79, y=w39) -> (x .and. y?=w271:bool)
  n441 = Not(x=w255) -> (.not. x?=w251:bool)
  n442 = Compound Arithmetic op=AND(w251, w248, w167) -> (w254:bool)
  n443 = Not(x=w254) -> (.not. x?=w250:bool)
  n444 = Bundle("OD"=w76, "OC"=w75, "OB"=w74, "OA"=w73, "OD"=w72, "OC"=w71, "OB"=w70, "OA"=w69) -> (→"W_reg":T17)  [unwired: 1 in]
  n445 = Not And(1:w283, 2:w282) -> (0:w281:bool)
  n446 = Not And(1:w281, 2:w154) -> (0:w260:bool)
  "WJ" <- w260
  n447 = And(x=w260, y=w260) -> (x .and. y?=w274:bool)
  n448 = Not And(1:w81, 2:w283) -> (0:w50:bool)
  "ADD" <- w50
  n449 = feedback #46() -> (w242:bool)  [unwired: 1 in]
  n450 = Compound Arithmetic op=AND(w242, w251, w250) -> (w256:bool)
  n451 = Not(x=w256) -> (.not. x?=w246:bool)
  n452 = Compound Arithmetic op=AND(w107, w107, w246) -> (w247:bool)
  n453 = Not(x=w247) -> (.not. x?=w244:bool)
  n454 = call "DflipFlop_Fast.vi"("D"=w244, "Clock"=w245, "Reset"=w257, "Set"=w257) -> ("/Q\\"=w37:bool, "Q"=w199:bool)  [unwired: 6 in]
  "ED" <- w37
  n455 = Not And(1:w199, 2:w630) -> (0:w625:bool)
  n456 = Compound Arithmetic op=AND(w625, w153, w135, w134) -> (w626:bool)
  n457 = Compound Arithmetic op=AND(w146, w150, w153, w625) -> (w631:bool)
  n458 = Not(x=w626) -> (.not. x?=w624:bool)
  n459 = Not(x=w631) -> (.not. x?=w629:bool)
  n460 = Not And(1:w624, 2:w624) -> (0:w565:bool)
  n461 = Not And(1:w629, 2:w629) -> (0:w563:bool)
  n462 = Compound Arithmetic op=AND(w584, w563, w581, w580, w557, w557, w148, w148) -> (w585:bool)
  n463 = Not(x=w585) -> (.not. x?=w546:bool)
  n464 = feedback-in #32(w546) -> ()
  n465 = Compound Arithmetic op=AND(w565, w565, w575, w574, w576, w576, w159, w155) -> (w579:bool)
  n466 = Not(x=w579) -> (.not. x?=w547:bool)
  n467 = feedback-in #31(w547) -> ()
  n468 = Compound Arithmetic op=AND(w564, w563, w567, w566, w565, w157, w563, w564) -> (w568:bool)
  n469 = Not(x=w568) -> (.not. x?=w549:bool)
  n470 = feedback-in #29(w549) -> ()
  n471 = feedback-in #46(w199) -> ()
  n472 = And(x=w305, y=w305) -> (x .and. y?=w309:bool)
  n473 = feedback #47() -> (w304:bool)  [unwired: 1 in]
  n474 = Not And(1:w315, 2:w304) -> (0:w314:bool)
  n475 = call "DflipFlop_Fast.vi"("D"=w314, "Clock"=w313, "Reset"=w317, "Set"=w317) -> ("/Q\\"=w51:bool, "Q"=w173:bool)  [unwired: 6 in]
  "C" <- w51
  n476 = Exclusive Or(1:w196, 2:w154) -> (0:w225:bool)
  n477 = feedback #48() -> (w237:bool)  [unwired: 1 in]
  n478 = Exclusive Or(1:w237, 2:TRUE ("x")) -> (0:w235:bool)
  n479 = feedback #49() -> (w234:bool)  [unwired: 1 in]
  n480 = feedback #50() -> (w229:bool)  [unwired: 1 in]
  n481 = Exclusive Or(1:w229, 2:TRUE ("x")) -> (0:w230:bool)
  n482 = Compound Arithmetic op=AND(w230, w137, w141) -> (w231:bool)
  n483 = Not(x=w231) -> (.not. x?=w227:bool)
  n484 = Not(x=w64) -> (.not. x?=w26:bool)
  n485 = Not(x=w63) -> (.not. x?=w27:bool)
  n486 = local read "Inputs"() -> (w18:T11)
  n487 = Unbundle By Name(w18) -> ("Init"=w17:bool)
  n488 = feedback #51() -> (w201:bool)  [unwired: 1 in]
  n489 = And(x=w201, y=w98) -> (x .and. y?=w435:bool)
  n490 = And(x=w97, y=w201) -> (x .and. y?=w434:bool)
  n491 = And(x=w201, y=w58) -> (x .and. y?=w471:bool)
  n492 = feedback #52() -> (w200:bool)  [unwired: 1 in]
  n493 = And(x=w200, y=w171) -> (x .and. y?=w470:bool)
  n494 = Not Or(1:w470, 2:w471) -> (0:w321:bool)
  n495 = Not And(1:w335, 2:w321) -> (0:w337:bool)
  n496 = Not And(1:w337, 2:w316) -> (0:w336:bool)
  n497 = Not And(1:w321, 2:w321) -> (0:w55:bool)
  "MR" <- w55
  n498 = And(x=w55, y=w99) -> (x .and. y?=w433:bool)
  n499 = Compound Arithmetic op=OR(w436, w435, w434, w433) -> (w432:bool)
  n500 = Not(x=w432) -> (.not. x?=w431:bool)
  n501 = Not And(1:w431, 2:w431) -> (0:w14:bool)
  n502 = call "7495_Fast2.vi"("Clk 1\nR-Shift"=w66, "Serial\nInput"=w14, "Clk 2\nL-Shift"=w66, "Mode\nControl"=w95, "D"=w440, "C"=w439, "B"=w438, "A"=w437) -> ("OD"=w13:bool, "OC"=w88:bool, "OB"=w87:bool, "OA"=w86:bool)
  "K4" <- w13
  "K5" <- w88
  "K6" <- w87
  "K7" <- w86
  n503 = feedback-in #10(w86) -> ()
  n504 = feedback-in #11(w87) -> ()
  n505 = feedback-in #12(w88) -> ()
  n506 = feedback-in #13(w13) -> ()
  n507 = call "7495_Fast2.vi"("Clk 1\nR-Shift"=w66, "Serial\nInput"=w13, "Clk 2\nL-Shift"=w66, "Mode\nControl"=w95, "D"=w441, "C"=w442, "B"=w443, "A"=w444) -> ("OD"=w19:bool, "OC"=w91:bool, "OB"=w90:bool, "OA"=w89:bool)
  "K0" <- w19
  "K1" <- w91
  "K2" <- w90
  "K3" <- w89
  n508 = feedback-in #19(w89) -> ()
  n509 = feedback-in #20(w90) -> ()
  n510 = feedback-in #21(w91) -> ()
  n511 = feedback-in #22(w19) -> ()
  n512 = Bundle("OD"=w19, "OC"=w91, "OB"=w90, "OA"=w89, "OD"=w13, "OC"=w88, "OB"=w87, "OA"=w86) -> (→"K_reg":T17)  [unwired: 1 in]
  n513 = call "DflipFlop_Fast.vi"("D"=w336, "Clock"=w313, "Reset"=w338, "Set"=w338) -> ("/Q\\"=w320:bool, "Q"=w40:bool)  [unwired: 6 in]
  "BD" <- w40
  n514 = feedback-in #36(w320) -> ()
  n515 = Compound Arithmetic op=AND(w320, w321, w249) -> (w331:bool)
  n516 = Compound Arithmetic op=AND(w318, w318, w55) -> (w330:bool)
  n517 = Compound Arithmetic op=AND(w83, w321, w40) -> (w333:bool)
  n518 = Not(x=w331) -> (.not. x?=w328:bool)
  n519 = Not(x=w330) -> (.not. x?=w329:bool)
  n520 = Not(x=w333) -> (.not. x?=w332:bool)
  n521 = Compound Arithmetic op=AND(w328, w332, w324, w329) -> (w334:bool)
  n522 = Not(x=w334) -> (.not. x?=w41:bool)
  "JC" <- w41
  n523 = Not And(1:w41, 2:w623) -> (0:w556:bool)
  n524 = Compound Arithmetic op=AND(w564, w556, w569, w139, w570, w138, w142, w141) -> (w573:bool)
  n525 = Not(x=w573) -> (.not. x?=w548:bool)
  n526 = feedback-in #30(w548) -> ()
  n527 = Compound Arithmetic op=AND(w560, w559, w557, w558, w150, w556, w148, w158) -> (w562:bool)
  n528 = Not(x=w562) -> (.not. x?=w198:bool)
  n529 = feedback-in #28(w198) -> ()
  n530 = Not And(1:w55, 2:w15) -> (0:w291:bool)
  n531 = Compound Arithmetic op=AND(w290, w289, w291) -> (w292:bool)
  n532 = Not(x=w292) -> (.not. x?=w288:bool)
  n533 = Compound Arithmetic op=AND(w354, w55, w345) -> (w362:bool)
  n534 = Not And(1:w282, 2:w288) -> (0:w286:bool)
  n535 = Not(x=w362) -> (.not. x?=w355:bool)
  n536 = Not And(1:w286, 2:w283) -> (0:w285:bool)
  n537 = Not And(1:w343, 2:w355) -> (0:w53:bool)
  "A" <- w53
  n538 = Not And(1:w284, 2:w285) -> (0:w170:bool)
  "WK" <- w170
  n539 = And(x=w170, y=w170) -> (x .and. y?=w277:bool)
  n540 = And(x=w170, y=w76) -> (x .and. y?=w268:bool)
  n541 = Compound Arithmetic op=OR(w277, w276, w275, w274) -> (w273:bool)
  n542 = Not(x=w273) -> (.not. x?=w261:bool)
  n543 = Not And(1:w261, 2:w261) -> (0:w57:bool)
  "WT" <- w57
  n544 = Exclusive Or(1:w53, 2:w50) -> (0:w298:bool)
  n545 = Not And(1:w298, 2:w298) -> (0:w300:bool)
  n546 = Exclusive Or(1:w239, 2:w55) -> (0:w240:bool)
  n547 = Compound Arithmetic op=AND(w240, w39, w78) -> (w241:bool)
  n548 = And(x=w173, y=w298) -> (x .and. y?=w306:bool)
  n549 = Not(x=w241) -> (.not. x?=w33:bool)
  "KP" <- w33
  n550 = Not And(1:w33, 2:w234) -> (0:w233:bool)
  n551 = Not And(1:w33, 2:w235) -> (0:w238:bool)
  n552 = Not And(1:w151, 2:w233) -> (0:w232:bool)
  n553 = call "7495_Fast2.vi"("Clk 1\nR-Shift"=w66, "Serial\nInput"=w226, "Clk 2\nL-Shift"=w66, "Mode\nControl"=w225, "D"=w227, "C"=w232, "B"=w238, "A"=w226) -> ("OD"=w32:bool, "OC"=w31:bool, "OB"=w30:bool)  [unwired: 1 out]
  "PO" <- w32
  "PT" <- w31
  "PF" <- w30
  n554 = And(x=w341, y=w32) -> (x .and. y?=w360:bool)
  n555 = Compound Arithmetic op=OR(w360, w359, w358, w357) -> (w356:bool)
  n556 = Not(x=w356) -> (.not. x?=w52:bool)
  "B" <- w52
  n557 = Not And(1:w52, 2:w52) -> (0:w299:bool)
  n558 = Exclusive Or(1:w52, 2:w53) -> (0:w312:bool)
  n559 = Exclusive Or(1:w173, 2:w312) -> (0:w49:bool)
  "SUM" <- w49
  n560 = And(x=w260, y=w49) -> (x .and. y?=w270:bool)
  n561 = Compound Arithmetic op=OR(w268, w269, w270, w271) -> (w272:bool)
  n562 = Not(x=w272) -> (.not. x?=w258:bool)
  n563 = Not And(1:w258, 2:w258) -> (0:w56:bool)
  "WD" <- w56
  n564 = feedback-in #45(w49) -> ()
  n565 = Compound Arithmetic op=AND(w300, w299, w173) -> (w303:bool)
  n566 = Compound Arithmetic op=AND(w298, w52, w51) -> (w302:bool)
  n567 = Not(x=w303) -> (.not. x?=w296:bool)
  n568 = Not(x=w302) -> (.not. x?=w297:bool)
  n569 = Compound Arithmetic op=AND(w296, w296, w297) -> (w301:bool)
  n570 = And(x=w52, y=w298) -> (x .and. y?=w307:bool)
  n571 = And(x=w52, y=w173) -> (x .and. y?=w308:bool)
  n572 = Not(x=w301) -> (.not. x?=w43:bool)
  "OF" <- w43
  n573 = call "DflipFlop_Fast.vi"("D"=w43, "Clock"=w293, "Reset"=w295, "Set"=w295) -> ("Q"=w47:bool)  [unwired: 6 in, 1 out]
  "OV" <- w47
  n574 = Compound Arithmetic op=OR(w306, w307, w308, w309) -> (w310:bool)
  n575 = Not(x=w310) -> (.not. x?=w45:bool)
  "CR" <- w45
  n576 = call "DflipFlop_Fast.vi"("D"=w45, "Clock"=w293, "Reset"=w294, "Set"=w294) -> ("Q"=w46:bool)  [unwired: 6 in, 1 out]
  "CY" <- w46
  n577 = feedback-in #47(w45) -> ()
  n578 = feedback-in #48(w30) -> ()
  n579 = feedback-in #49(w31) -> ()
  n580 = feedback-in #50(w32) -> ()
  n581 = Not And(1:w47, 2:w125) -> (0:w213:bool)
  n582 = Not And(1:w46, 2:w124) -> (0:w212:bool)
  n583 = Not And(1:w171, 2:w57) -> (0:w221:bool)
  n584 = Not And(1:w58, 2:w57) -> (0:w215:bool)
  n585 = Not And(1:w212, 2:w213) -> (0:w214:bool)
  n586 = Bundle(w53, w52, "/Q\\"=w51, w50, w49, "/Q\\"=w48, "Q"=w47, "Q"=w46, w45, w44, w43) -> (→"Adder":T18)  [unwired: 1 in]
  n587 = Not And(1:w214, 2:w48) -> (0:w211:bool)
  n588 = Not And(1:w221, 2:w221) -> (0:w224:bool)
  n589 = Not And(1:w215, 2:w215) -> (0:w218:bool)
  n590 = Compound Arithmetic op=AND(w176, w201, w215, w208) -> (w217:bool)
  n591 = Not And(1:w56, 2:w224) -> (0:w223:bool)
  n592 = Not And(1:w200, 2:w221) -> (0:w222:bool)
  n593 = Not(x=w217) -> (.not. x?=w216:bool)
  n594 = Not And(1:w56, 2:w218) -> (0:w219:bool)
  n595 = Not And(1:w222, 2:w223) -> (0:w62:bool)
  "JDL0" <- w62
  n596 = Compound Arithmetic op=AND(w216, w211, w219, w206) -> (w220:bool)
  n597 = Not(x=w220) -> (.not. x?=w61:bool)
  "JDL1" <- w61
  n598 = Bundle("Clk"=w67, w66, w65, w64, w63, w62, w61, w60, w59, "/Q\\"=w58, w57, w56, w55) -> (→"Clocks And Memory":T19)  [unwired: 1 in]
  n599 = Bundle(w41, "Q"=w40, w39, w38, "/Q\\"=w37, w36, w35, "OD"=w34, w33, "OD"=w32, "OC"=w31, "OB"=w30) -> (→"Instruction Specific":T20)  [unwired: 1 in]
  n600 = Not And(1:w62, 2:w62) -> (0:w28:bool)
  n601 = Not And(1:w61, 2:w61) -> (0:w205:bool)
  n602 = case shown="False" FALSE {
    tunnel: w205 -> [w678 w687]
    tunnel: [w681 w686] -> w24
    tunnel: [w679 w685] -> w23
    tunnel: w28 -> [w680 w684]
    tunnel: w27 -> [w675 w683]
    tunnel: w26 -> [w676 w682]
    tunnel: w17 -> [w677 _]
    tunnel: w16 -> [w674 _]
    frame False {
      n603 = call "Mem1024_Fast2.vi"("Reset"=w674, "Init"=w677, "Phi2"=w675, "Phi1"=w676, "In"=w680) -> ("Out"=w681:bool)  [unwired: 5 in, 1 out]
      n604 = call "Mem1024_Fast2.vi"("Reset"=w674, "Init"=w677, "Phi2"=w675, "Phi1"=w676, "In"=w678) -> ("Out"=w679:bool)  [unwired: 5 in, 1 out]
    }
    frame True {
      n605 = call "Mem1024.vi"("Phi2"=w683, "Phi1"=w682, "Data In"=w684) -> ("Data Out"=w686:bool)  [unwired: 8 in]
      n606 = call "Mem1024.vi"("Phi2"=w683, "Phi1"=w682, "Data In"=w687) -> ("Data Out"=w685:bool)  [unwired: 8 in]
    }
  }
  n607 = Not And(1:w24, 2:w204) -> (0:w203:bool)
  n608 = feedback-in #52(w203) -> ()
  n609 = Not And(1:w23, 2:w204) -> (0:w202:bool)
  n610 = feedback-in #51(w202) -> ()
  n611 = call "Mem2Num.vi"("Reset"=w16, "Data In"=w23) -> ("Mem"=w21:u8)  [unwired: 9 in]
  n612 = call "Mem2Num.vi"("Reset"=w16, "Data In"=w24) -> ("Mem"=w22:u8)  [unwired: 9 in]
  n613 = Bundle("Mem"=w22, "Mem"=w21, w16) -> (→"Memory":cluster{"Mem":u8, "Mem":u8, bool})  [unwired: 1 in]
